vi "encoder_test_3mode_2motor_v3.vi"() -> ()   [LabVIEW 2014]
uses:
  <vilib>/rvi/FXPMathLib/FxpSinAndCos/subVIs/nifxpmath_SinAndCos_SimConfig.ctl
  <vilib>/rvi/Emulation/niFpgaGetClockAttributes.vi
  <vilib>/rvi/Emulation/niFpgaSctlEmulationGetInTimedLoop.vi
  <vilib>/rvi/Emulation/niFpgaEmulationReportErrorSimple.vi
  <vilib>/rvi/eio/common/nirviEmuTemplateMethod_errors.vi
  <vilib>/rvi/Emulation/niFpgaProcessEmulError.vi
  <vilib>/rvi/Emulation/niFpgaCriticalErrorInLSC.vi
  <vilib>/rvi/FXPMathLib/FxpSinAndCos/simVIs/DllFxpSinAndCosTemp_sub.vi
  <vilib>/rvi/interface/RandomDataEmulation/nirviRandomDataMultiElementFPGAFIFO.vi
  <instcachedir>/0/nirviRandomDataMultiElementFPGAFIFO_AD0CFC12EF974623A9C2E4184BC062B2.lvgen/nirviRandomDataMultiElementFPGAFIFO_AD0CFC12EF974623A9C2E4184BC062B2_020.vi
  <vilib>/rvi/interface/RandomDataEmulation/niFpgaRandomDataHandleErrors.vi
  <vilib>/eio/EIONode/EIONode.xnode
  <vilib>/rvi/FXPMathLib/FxpMul/XNode/nifxpmath_Multiplier.xnode
  <vilib>/rvi/FXPMathLib/FxpSinAndCos/XNode/nifxpmath_SinAndCos.xnode
  <vilib>/rvi/Analysis/measure/butterworth/XNode/niFpgaButterworthFilter.xnode
  <vilib>/rvi/FXPMathLib/FxpSub/XNode/nifxpmath_Sub.xnode
  <vilib>/rvi/FXPMathLib/FxpAdd/XNode/nifxpmath_Add.xnode
  <vilib>/rvi/DataTransferAndStorage/Container/XNode/niFpgaContainer.xnode
  <vilib>/rvi/interface/RandomDataEmulation/nirviRandomDataFpgaMultiElementTemplate.vi
  <vilib>/rvi/FXPMathLib/sim/FxpSim.dll
panel:
  out "Dyr_sin_dd":fxp<+/-,64,25>
  out "Dyr_sin_d":fxp<+/-,64,16>
  out "Dyr_sin":fxp<+/-,30,11>
  in  "Sin offset_y":fxp<+/-,29,10>
  out "Sin omega_y":fxp<+/-,41,8>
  in  "Sin magnitude_y":fxp<+/-,11,8>
  in  "Sin wave frequency_y (Hz)":fxp<+/-,21,5>
  out "Dyr_ramp":fxp<+/-,32,7>
  out "Time now_y (s)":fxp<+,52,14>
  out "Dyr_slope":fxp<+/-,32,10>
  in  "Dyr_time":fxp<+/-,32,10>
  in  "Dyr_end":fxp<+/-,32,7>
  out "Dy_i":fxp<+/-,32,16>
  out "Dyr":fxp<+/-,32,7>
  in  "Direction_y":bool
  in  "Command type_y":i16(ring) items=["Step", "Ramp", "Sine"]
  out "Dy_error":fxp<+/-,57,33>
  out "Fmr_y":fxp<+/-,64,50>
  in  "Ki_y":fxp<+/-,16,1>
  in  "Dy_tolorence":fxp<+/-,18,1>
  in  "Kd_y":fxp<+/-,16,1>
  in  "Kp_y":fxp<+/-,16,1>
  in  "scaled coefficients_Dy_dd":i32[](array[numeric])=[780119100, 146811362]
  out "Dy_dd":fxp<+/-,36,47>
  out "va_y":fxp<+/-,36,7>
  out "vb_y":fxp<+/-,37,8>
  out "vd_y":fxp<+/-,20,5>
  out "vq_y":fxp<+/-,20,5> format="%.57g"
  in  "Stop motor_y":bool
  out "Dy_d (mm/s)":fxp<+,64,32>
  out "omega_y (rad/s)":fxp<+/-,64,35>
  in  "Velocity Estimation_y":i16(ring) items=["Step", "Ramp", "Sine"]
  out "Dy_d (T)":fxp<+/-,46,10>
  out "mt 2":u32
  out "omega_y (T)":fxp<+/-,20,9>
  out "omega_y (M)":fxp<+/-,64,30>
  out "Dy_d (M)":fxp<+/-,64,27>
  in  "Dy_d_M_Tc (mSec)":u32 format="%#_6f"
  out "omega_y(M_avg)":fxp<+/-,64,35>
  out "Dy_d (M_avg)":fxp<+,64,32>
  in  "Dy_d_M_avg_Tc (uSec)":u32 caption="Count(uSec)"
  out "rad_y(NrTheta)":fxp<+/-,48,33>
  out "Dy (mm)":fxp<+/-,56,32>
  out "Encoder Position_y":i32
  in  "Encoder Reset_y":bool
  out "omega_p (M_avg)":fxp<+/-,64,35>
  out "Dp_d (M_avg)":fxp<+/-,64,32>
  in  "Dp_d_M_avg_Tc (uSec)":u32 caption="D_d_M_avg_Tc (uSec)"
  out "omega_p (M)":fxp<+/-,64,30>
  out "Dp_d (M)":fxp<+/-,64,27>
  in  "Dp_d_M_Tc (mSec)":u32 format="%#_6f"
  out "Dp_d (T)":fxp<+/-,46,10>
  out "omega_p(T)":fxp<+/-,20,9>
  in  "Velocity Estimation_p":i16(ring) items=["M_avg method", "M method", "T method"]
  out "Dpr_ramp":fxp<+/-,64,30>
  out "Dpr_slope":fxp<+/-,32,10>
  in  "Dpr_time":fxp<+/-,32,10>
  out "Dpr_sin":fxp<+/-,30,11>
  out "Dpr_sin_d":fxp<+/-,64,16>
  out "Dpr_sin_dd":fxp<+/-,64,25>
  out "Sin omega_p":fxp<+/-,41,8>
  in  "Sin offset_p":fxp<+/-,27,10>
  in  "Sin magnitude_p":fxp<+/-,11,8>
  in  "Sin wave frequency_p (Hz)":fxp<+/-,21,5>
  out "Time now_p (s)":fxp<+,52,14>
  out "Dpr":fxp<+/-,64,31>
  in  "Dpr_end":fxp<+/-,22,7>
  in  "Command type_p":i16(ring) items=["Step", "Ramp", "Sine"]
  out "Dp_i":fxp<+/-,34,18>
  in  "Dp_tolorence":fxp<+/-,18,1>
  in  "Ki_p":fxp<+/-,20,6>
  out "Dp_error":fxp<+/-,24,11>
  in  "Direction_p":bool
  out "Fmr_p":fxp<+/-,64,31>
  in  "Kd_p":fxp<+/-,20,8>
  in  "Kp_p":fxp<+/-,20,12>
  in  "scaled coefficients_Dp_dd":i32[](array[numeric])=[780119100, 146811362]
  out "Dp_dd":fxp<+/-,36,29>
  in  "Ini coe.":bool
  out "va_p":fxp<+/-,38,8>
  out "vb_p":fxp<+/-,38,8>
  in  "Stop motor_p":bool
  out "vq_p":fxp<+/-,20,5> format="%.57g"
  out "vd_p":fxp<+/-,20,5>
  out "Dp_d (mm/s)":fxp<+/-,32,12>
  out "mt":u32
  out "omega_p (rad/s)":fxp<+/-,32,18>
  in  "mt0":u32
  out "Dp (mm)":fxp<+/-,22,7>
  out "rad_p(NrTheta)":fxp<+/-,33,18>
  out "Encoder Position_p":i32
  in  "Encoder Reset_p":bool
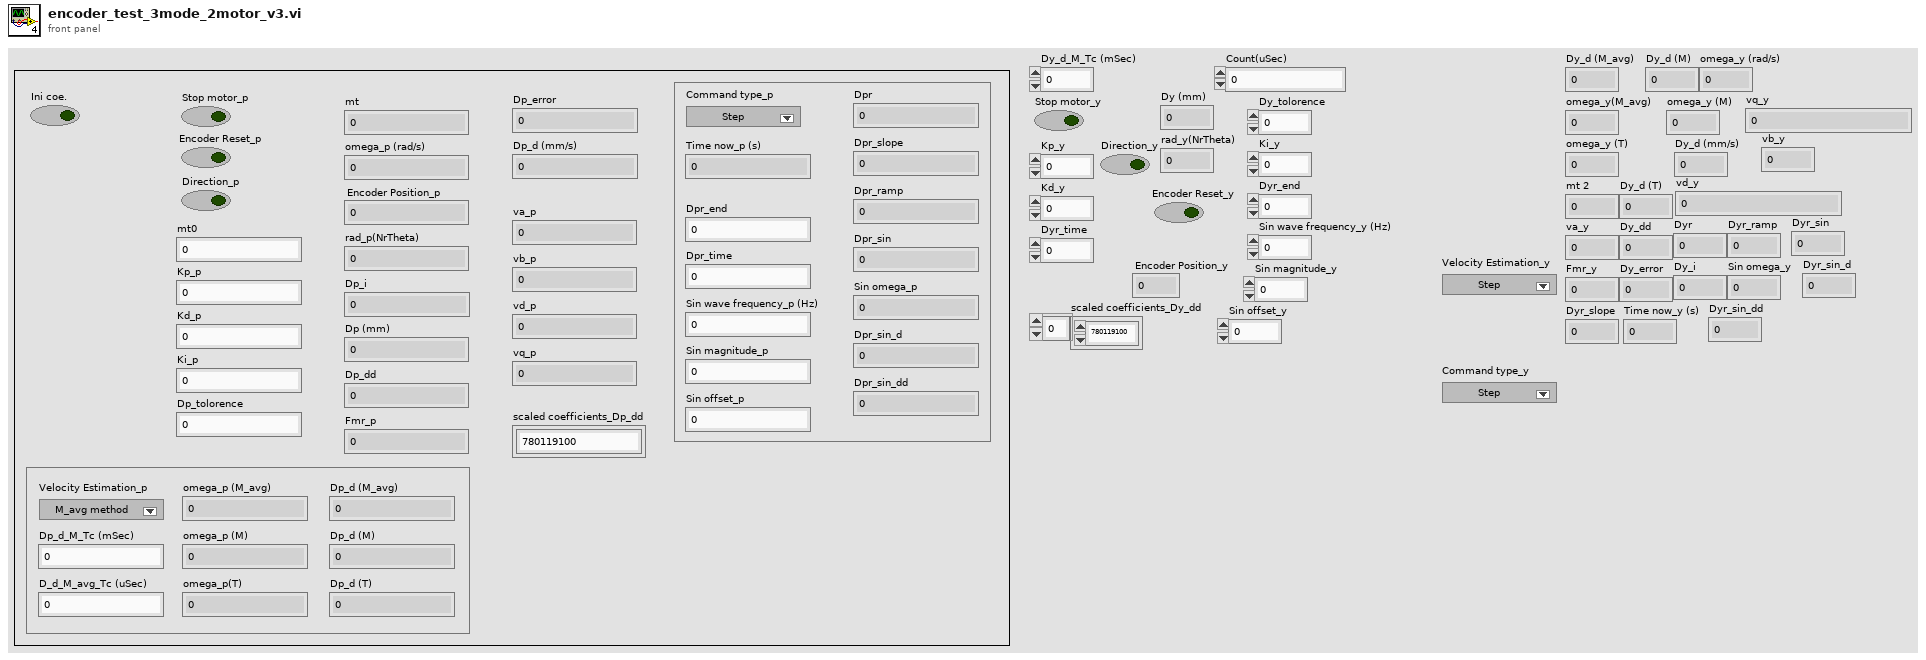
[diagram p1: front panel]
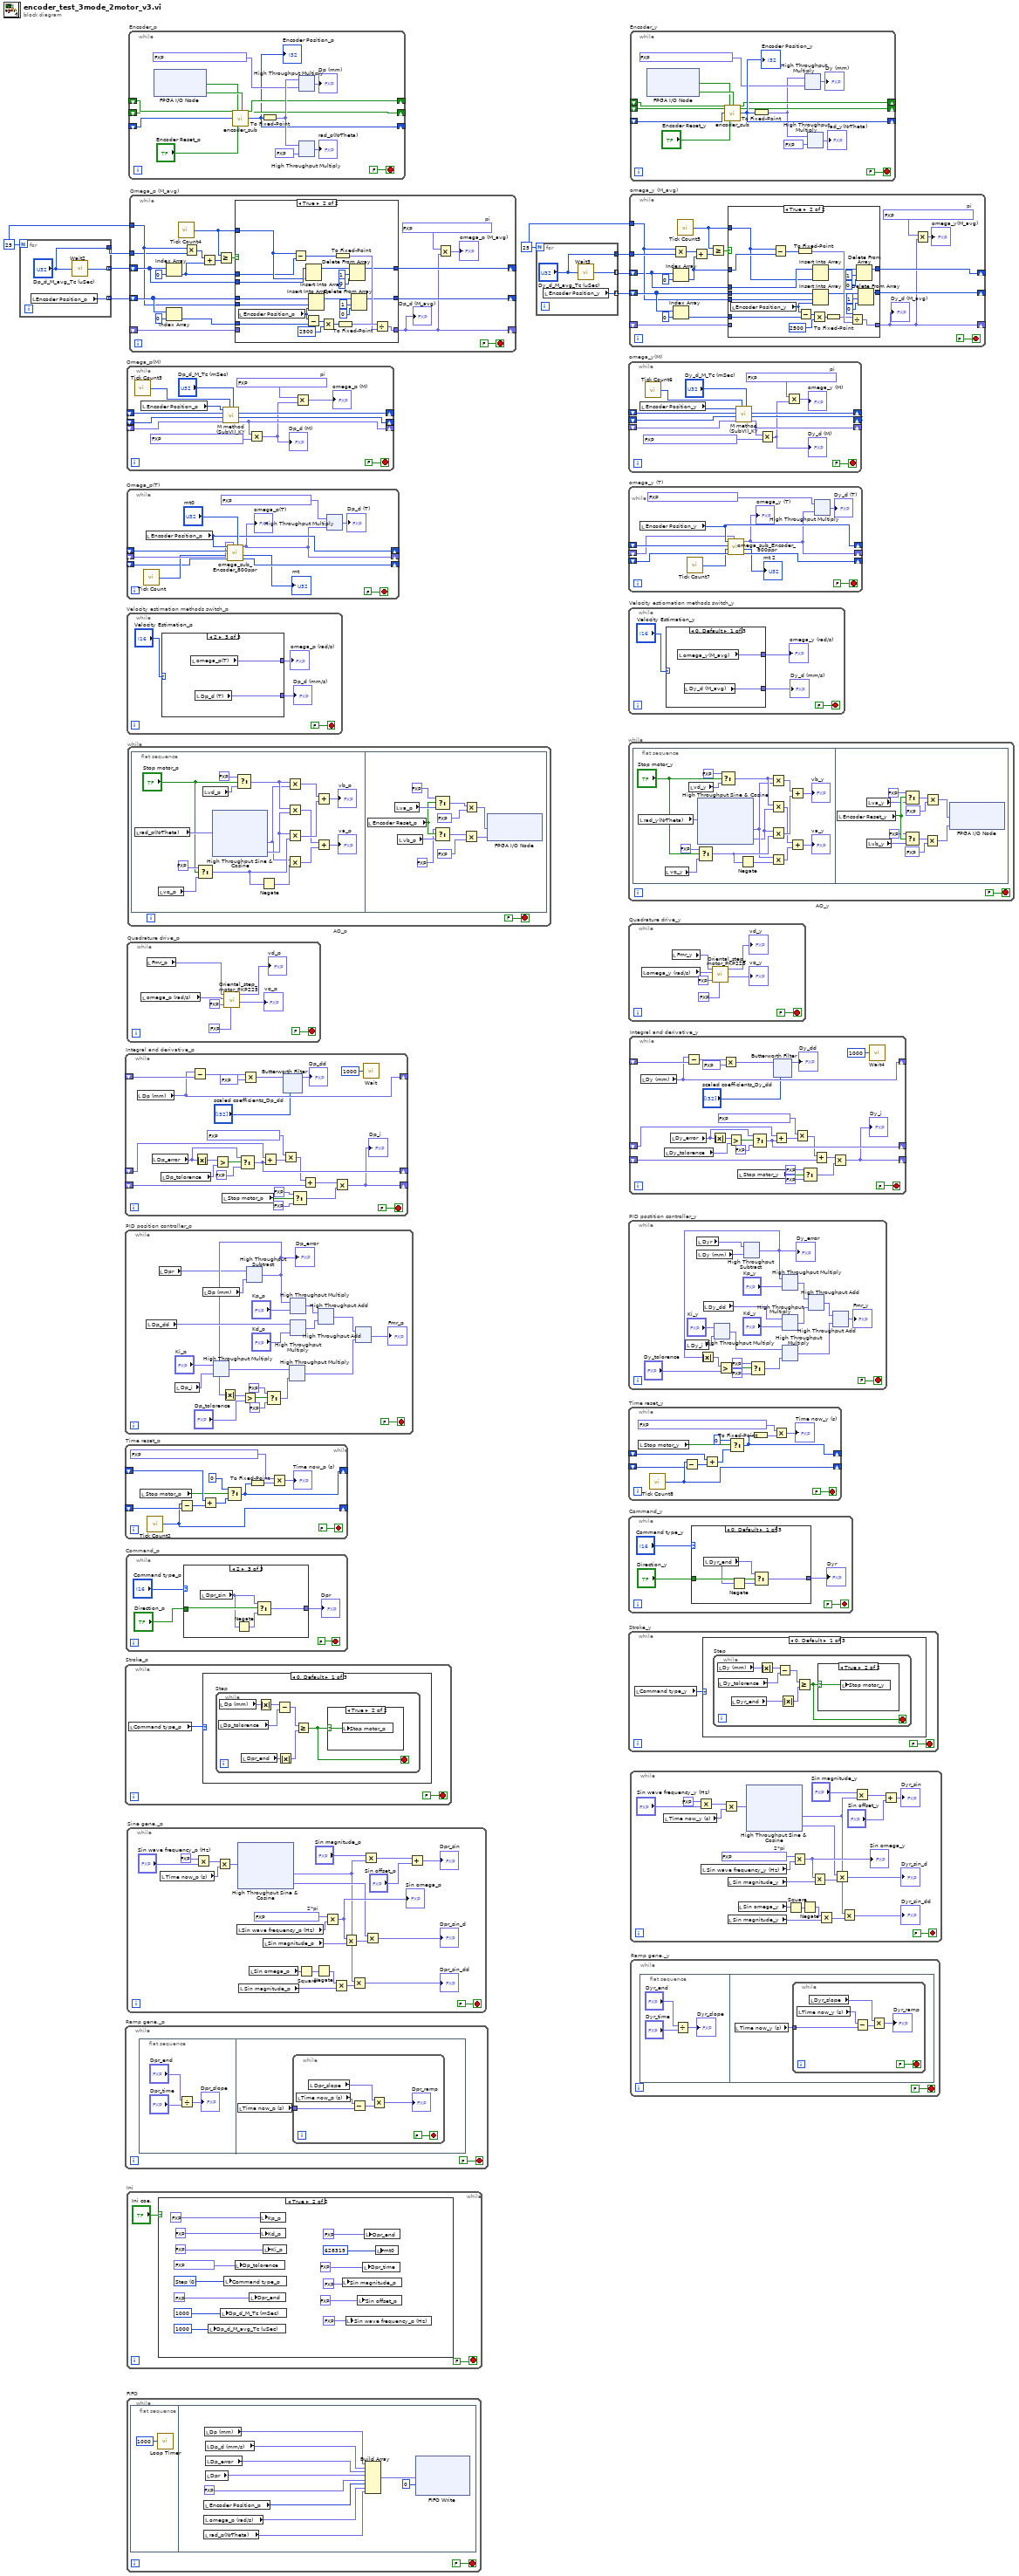
[diagram p0: block diagram]
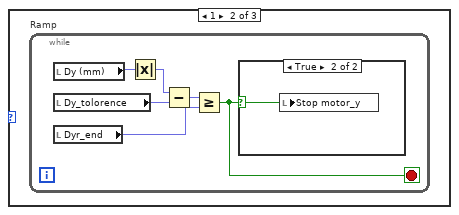
[diagram p3: hidden frame]
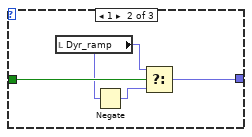
[diagram p6: hidden frame]
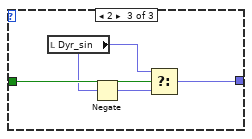
[diagram p7: hidden frame]
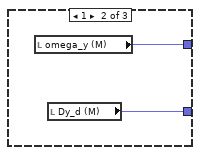
[diagram p8: hidden frame]
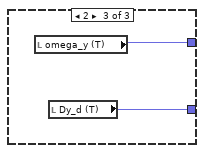
[diagram p9: hidden frame]
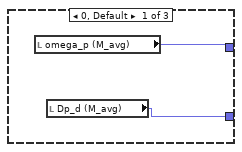
[diagram p12: hidden frame]
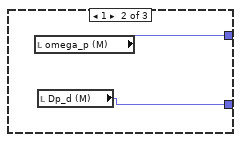
[diagram p13: hidden frame]
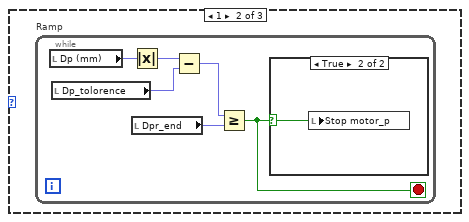
[diagram p15: hidden frame]
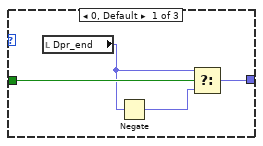
[diagram p18: hidden frame]
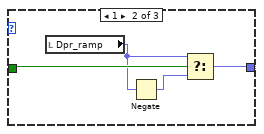
[diagram p19: hidden frame]
diagram:
  w4 = 25
  w8 = 25
  n1 = for {
    N: w8 -> [_]
    tunnel: ["Dp_d_M_avg_Tc (uSec)"] -> w5
    tunnel: [w10] -> w7 mode=indexing
    tunnel: [w9] -> w6 mode=indexing
    n2 = local read "Encoder Position_p"() -> (w9:i32)
    n3 = call "Wait2"("Count(uSec)"="Dp_d_M_avg_Tc (uSec)") -> ("Tick Count(uSec)"=w10:u32)
  }
  n4 = while "Integral and derivative_p" {
    shift-right: [w32] -> _
    shift-left: _ -> [w36]
    shift-right: [w22] -> _
    shift-left: _ -> [w23]
    shift-right: [w12] -> _
    shift-left: _ -> [w16]
    stop <- FALSE stop-if-true
    n5 = local read "Dp (mm)"() -> (w32:fxp<+/-,22,7>)
    n6 = local read "Dp_error"() -> (w24:fxp<+/-,24,11>)
    n7 = local read "Dp_tolorence"() -> (w27:fxp<+/-,18,1>)
    n8 = Subtract(x=w32, y=w36) -> (x-y=w35:fxp<+/-,23,8>)
    n9 = Absolute Value(x=w24) -> (abs(x)=w28:fxp<+,24,11>)
    n10 = Greater?(x=w28, y=w27) -> (0:w26:bool)
    n11 = local read "Stop motor_p"() -> (w19:bool)
    n12 = Select(t=w24, s=w26, f=fxp<+,24,11> 0.0) -> (s? t:f=w22:fxp<+/-,25,12>)
    n13 = Multiply(x=w35, y=fxp<+/-,33,13> 1000.0) -> (x*y=w33:fxp<+/-,55,20>)
    n14 = Add(x=w23, y=w22) -> (x+y=w21:fxp<+/-,26,13>)
    n15 = Multiply(x=fxp<+/-,30,12> 0.000499725341796875, y=w21) -> (x*y=w15:fxp<+/-,55,24>)
    n16 = xnode "Butterworth Filter"("input data"=w33, "scaled coefficients"="scaled coefficients_Dp_dd") -> ("output data"=→"Dp_dd":fxp<+/-,36,24>)  [unwired: 1 in]
    n17 = Select(t=fxp<+,1,1> 0.0, s=w19, f=fxp<+,1,1> 1.0) -> (s? t:f=w13:fxp<+,1,1>)
    n18 = Add(x=w15, y=w16) -> (x+y=w14:fxp<+/-,32,16>)
    n19 = Multiply(x=w14, y=w13) -> (x*y=w12:fxp<+/-,32,16>)
    "Dp_i" <- w12
    n20 = call "Wait"("Count(uSec)"=u32 1000) -> ()  [unwired: 1 out]
  }
  n21 = while "PID position controller_p" {
    stop <- FALSE stop-if-true
    n22 = local read "Dp_dd"() -> (w62:fxp<+/-,36,29>)
    n23 = local read "Dpr"() -> (w46:fxp<+/-,64,31>)
    n24 = local read "Dp_i"() -> (w57:fxp<+/-,34,18>)
    n25 = local read "Dp (mm)"() -> (w66:fxp<+/-,22,7>)
    n26 = xnode ("High Throughput Multiply")("x"="Ki_p", "y"=w57) -> ("x*y"=w51:fxp<+/-,54,24>)
    n27 = xnode "High Throughput Subtract"("x"=w46, "y"=w66) -> ("x-y"=w55:fxp<+/-,64,32>)
    "Dp_error" <- w55
    n28 = Absolute Value(x=w55) -> (abs(x)=w56:fxp<+,64,32>)
    n29 = Greater?(x=w56, y="Dp_tolorence") -> (0:w54:bool)
    n30 = Select(t=fxp<+,10,2> 1.0, s=w54, f=fxp<+,10,2> 0.0) -> (s? t:f=w50:fxp<+,10,2>)
    n31 = xnode ("High Throughput Multiply")("x"=w51, "y"=w50) -> ("x*y"=w47:fxp<+/-,64,26>)
    n32 = xnode ("High Throughput Multiply")("x"=w55, "y"="Kp_p") -> ("x*y"=w64:fxp<+/-,64,44>)
    n33 = xnode ("High Throughput Multiply")("x"=w62, "y"="Kd_p") -> ("x*y"=w63:fxp<+/-,56,37>)
    n34 = xnode ("High Throughput Add")("x"=w64, "y"=w63) -> ("x+y"=w48:fxp<+/-,64,45>)
    n35 = xnode ("High Throughput Add")("x"=w48, "y"=w47) -> ("x+y"=→"Fmr_p":fxp<+/-,64,46>)
  }
  n36 = while "Time reset_p" {
    shift-right: [w70] -> _
    shift-left: _ -> [w77]
    shift-right: [w72] -> _
    shift-left: _ -> [w73]
    stop <- FALSE stop-if-true
    n37 = local read "Stop motor_p"() -> (w75:bool)
    n38 = call "Tick Count2"() -> ("Tick Count(uSec)"=w72:u32)
    n39 = Subtract(x=w72, y=w73) -> (x-y=w78:u32)
    n40 = Add(x=w77, y=w78) -> (x+y=w76:u32)
    n41 = Select(t=u32 0, s=w75, f=w76) -> (s? t:f=w70:u32)
    n42 = To Fixed-Point(number=w70) -> (fixed-point=w69:fxp<+,32,32>)  [unwired: 1 in]
    n43 = Multiply(x=fxp<+,20,-18> 1.0000003385357559e-06, y=w69) -> (x*y=→"Time now_p (s)":fxp<+,52,14>)
  }
  n44 = while "Stroke_p" {
    stop <- FALSE stop-if-true
    n45 = local read "Command type_p"() -> (w80:i16)
    n46 = case shown="0, Default" w80 {
      frame 0, Default {
        n47 = while "Step" {
          stop <- w81 stop-if-true
          n48 = local read "Dp_tolorence"() -> (w83:fxp<+/-,18,1>)
          n49 = local read "Dp (mm)"() -> (w85:fxp<+/-,22,7>)
          n50 = local read "Dpr_end"() -> (w87:fxp<+/-,22,7>)
          n51 = Absolute Value(x=w85) -> (abs(x)=w84:fxp<+,22,7>)
          n52 = Subtract(x=w84, y=w83) -> (x-y=w82:fxp<+/-,25,8>)
          n53 = Absolute Value(x=w87) -> (abs(x)=w86:fxp<+,22,7>)
          n54 = Greater Or Equal?(x=w82, y=w86) -> (x >= y?=w81:bool)
          n55 = case shown="True" w81 {
            selector: w81 -> [_ w88]
            frame False {
            }
            frame True {
              n56 = local write "Stop motor_p"(w88) -> ()
            }
          }
        }
      }
      frame 1 {
        n57 = while "Ramp" {
          stop <- w89 stop-if-true
          n58 = local read "Dp (mm)"() -> (w91:fxp<+/-,22,7>)
          n59 = local read "Dp_tolorence"() -> (w93:fxp<+/-,18,1>)
          n60 = Absolute Value(x=w91) -> (abs(x)=w92:fxp<+,22,7>)
          n61 = local read "Dpr_end"() -> (w90:fxp<+/-,22,7>)
          n62 = Subtract(x=w92, y=w93) -> (x-y=w94:fxp<+/-,25,8>)
          n63 = Greater Or Equal?(x=w94, y=w90) -> (x >= y?=w89:bool)
          n64 = case shown="True" w89 {
            selector: w89 -> [_ w95]
            frame False {
            }
            frame True {
              n65 = local write "Stop motor_p"(w95) -> ()
            }
          }
        }
      }
      frame 2 {
      }
    }
  }
  n66 = while "Ramp gene._p" {
    stop <- FALSE stop-if-true
    n67 = flat-sequence {
      frame #0 {
        n68 = Divide(x="Dpr_end", y="Dpr_time") -> (x/y=→"Dpr_slope":fxp<+/-,55,30>)
      }
      frame #1 {
        n69 = local read "Time now_p (s)"() -> (w100:fxp<+,52,14>)
        n70 = while {
          tunnel: w100 -> [w106]
          stop <- FALSE stop-if-true
          n71 = local read "Time now_p (s)"() -> (w103:fxp<+,52,14>)
          n72 = local read "Dpr_slope"() -> (w104:fxp<+/-,32,10>)
          n73 = Subtract(x=w103, y=w106) -> (x-y=w105:fxp<+/-,53,15>)
          n74 = Multiply(x=w104, y=w105) -> (x*y=→"Dpr_ramp":fxp<+/-,64,24>)
        }
      }
    }
  }
  n75 = while "Command_p" {
    stop <- FALSE stop-if-true
    n76 = case shown="2" "Command type_p" {
      tunnel: [w111 w115 w119] -> w109
      tunnel: "Direction_p" -> [w114 w118 w122]
      frame 0, Default {
        n77 = local read "Dpr_end"() -> (w113:fxp<+/-,22,7>)
        n78 = Negate(x=w113) -> (-x=w112:fxp<+/-,23,8>)
        n79 = Select(t=w113, s=w114, f=w112) -> (s? t:f=w111:fxp<+/-,23,8>)
      }
      frame 1 {
        n80 = local read "Dpr_ramp"() -> (w116:fxp<+/-,64,30>)
        n81 = Negate(x=w116) -> (-x=w117:fxp<+/-,64,31>)
        n82 = Select(t=w116, s=w118, f=w117) -> (s? t:f=w115:fxp<+/-,64,31>)
      }
      frame 2 {
        n83 = local read "Dpr_sin"() -> (w120:fxp<+/-,30,11>)
        n84 = Negate(x=w120) -> (-x=w121:fxp<+/-,29,10>)
        n85 = Select(t=w120, s=w122, f=w121) -> (s? t:f=w119:fxp<+/-,30,11>)
      }
    }
    "Dpr" <- w109
  }
  n86 = while "Omega_p(M)" {
    shift-right: [w134] -> _
    shift-left: _ -> [w135]
    shift-right: [w130] -> _
    shift-left: _ -> [w131]
    shift-right: [w128] -> _
    shift-left: _ -> [w129]
    stop <- FALSE stop-if-true
    w125 = fxp<+/-,27,3> 3.1415926218032837  # pi
    n87 = call "Tick Count3"() -> ("Tick Count(mSec)"=w133:u32)
    n88 = local read "Encoder Position_p"() -> (w136:i32)
    n89 = call "M method (SubVI)_KY.vi"("Tc (mSec)"="Dp_d_M_Tc (mSec)", "Tick Count (mSec)"=w133, "Encoder velocity_pre (pulse/s)"=w129, "Shift Register in 2"=w131, "Shift Register in 1"=w135, "Encoder pulses"=w136) -> ("Encoder velocity (pulse/s)"=w128:fxp<+/-,64,32>, "Shift Register out 2"=w130:i32, "Shift Register out 1"=w134:u32)  [unwired: 3 in]
    n90 = Multiply(x=w128, y=fxp<+/-,20,-5> 0.002499997615814209) -> (x*y=w126:fxp<+/-,64,27>)
    "Dp_d (M)" <- w126
    n91 = Multiply(x=w125, y=w126) -> (x*y=→"omega_p (M)":fxp<+/-,64,30>)
  }
  n92 = while "Omega_p(T)" {
    shift-right: [w146] -> _
    shift-left: _ -> [w147]
    shift-right: [w139] -> _
    shift-left: _ -> [w145]
    shift-right: [w142] -> _
    shift-left: _ -> [w143]
    stop <- FALSE stop-if-true
    n93 = call "Tick Count"() -> ("Tick Count(Ticks)"=w144:u32)
    n94 = local read "Encoder Position_p"() -> (w146:i32)
    n95 = call "omega_sub_Encoder_800ppr.vi"("mt0"="mt0", "omega_pre"=w145, "ticks_m_pre"=w143, "ticks"=w144, "count_pre"=w147, "count"=w146) -> ("ticks_m"=w142:u32, "mt"=→"mt":u32, "omega"=w139:fxp<+/-,20,9>)  [unwired: 3 in]
    "omega_p(T)" <- w139
    n96 = xnode ("High Throughput Multiply")("x"=fxp<+/-,26,1> 0.3183099031448364, "y"=w139) -> ("x*y"=→"Dp_d (T)":fxp<+/-,46,10>)
  }
  n97 = while "Velocity estimation methods switch_p" {
    stop <- FALSE stop-if-true
    n98 = case shown="2" "Velocity Estimation_p" {
      tunnel: [w154 w156 w158] -> w151
      tunnel: [w153 w155 w157] -> w150
      frame 0, Default {
        n99 = local read "omega_p (M_avg)"() -> (w154:fxp<+/-,64,35>)
        n100 = local read "Dp_d (M_avg)"() -> (w153:fxp<+/-,64,32>)
      }
      frame 1 {
        n101 = local read "omega_p (M)"() -> (w156:fxp<+/-,64,30>)
        n102 = local read "Dp_d (M)"() -> (w155:fxp<+/-,64,27>)
      }
      frame 2 {
        n103 = local read "omega_p(T)"() -> (w158:fxp<+/-,20,9>)
        n104 = local read "Dp_d (T)"() -> (w157:fxp<+/-,46,10>)
      }
    }
    "Dp_d (mm/s)" <- w150
    "omega_p (rad/s)" <- w151
  }
  n105 = while "Ini" {
    stop <- FALSE stop-if-true
    n106 = case shown="True" "Ini coe." {
      frame False {
      }
      frame True {
        w168 = i16 0 items=["Step", "Ramp", "Sine"] ("Command type")
        n107 = local write "Dp_d_M_avg_Tc (uSec)"(u32 1000 ("D_d_M_avg_Tc (uSec)")) -> ()
        n108 = local write "Dp_d_M_Tc (mSec)"(u32 1000 ("D_d_M_Tc (uSec)")) -> ()
        n109 = local write "Command type_p"(w168) -> ()
        n110 = local write "Dp_tolorence"(fxp<+/-,14,3> 0.009765625 ("D_tolorence")) -> ()
        n111 = local write "Dpr_end"(fxp<+/-,16,11> 20.0 ("Dr_end")) -> ()
        n112 = local write "Kp_p"(fxp<+/-,20,12> 10.0 ("Kp")) -> ()
        n113 = local write "Kd_p"(fxp<+/-,20,8> 2.0 ("Kd")) -> ()
        n114 = local write "Ki_p"(fxp<+/-,20,6> 8.0 ("D_i")) -> ()
        n115 = local write "Sin magnitude_p"(fxp<+/-,11,8> 20.0 ("Sin magnitude")) -> ()
        n116 = local write "Sin wave frequency_p (Hz)"(fxp<+/-,21,5> 0.5 ("Sin wave frequency (Hz)")) -> ()
        n117 = local write "Sin offset_p"(fxp<+/-,27,10> 0.0 ("Sin offset")) -> ()
        n118 = local write "Dpr_time"(fxp<+/-,16,11> 5.0 ("Dr_time")) -> ()
        n119 = local write "Dpr_end"(fxp<+/-,11,7> 20.0 ("Fmr")) -> ()
        n120 = local write "mt0"(u32 628319 ("mt0")) -> ()
      }
    }
  }
  n121 = while "FIFO" {
    stop <- FALSE stop-if-true
    n122 = flat-sequence {
      frame #0 {
        n123 = call "Loop Timer"("Count(uSec)"=u32 1000) -> ()  [unwired: 1 out]
      }
      frame #1 {
        n124 = local read "Encoder Position_p"() -> (w180:i32)
        n125 = local read "omega_p (rad/s)"() -> (w179:fxp<+/-,32,18>)
        n126 = local read "rad_p(NrTheta)"() -> (w178:fxp<+/-,33,18>)
        n127 = local read "Dp (mm)"() -> (w184:fxp<+/-,22,7>)
        n128 = local read "Dp_d (mm/s)"() -> (w183:fxp<+/-,32,12>)
        n129 = local read "Dp_error"() -> (w182:fxp<+/-,24,11>)
        n130 = local read "Dpr"() -> (w181:fxp<+/-,64,31>)
        n131 = Build Array(w184, w183, w182, w181, fxp<+/-,64,32> 0.0 ("element"), w180, w179, w178) -> (w185:fxp<+/-,64,32>[])
        n132 = xnode ("FIFO Write")("Element"=w185, "Timeout"=0) -> ()  [unwired: 1 in, 2 out]
      }
    }
  }
  n133 = while "Quadrature drive_p" {
    stop <- FALSE stop-if-true
    n134 = local read "omega_p (rad/s)"() -> (w189:fxp<+/-,32,18>)
    n135 = local read "Fmr_p"() -> (w187:fxp<+/-,64,31>)
    n136 = call "Oriental_step_motor_PKP225.vi"("F_Threshold"=fxp<+,12,12> 10.0, "dFmr"=fxp<+/-,25,15> 0.0, "omega"=w189, "Fmr"=w187) -> ("vq_F"=→"vq_p":fxp<+/-,20,5>, "vd_F"=→"vd_p":fxp<+/-,20,5>)  [unwired: 6 in]
  }
  n137 = while "Sine gene._p" {
    stop <- FALSE stop-if-true
    w211 = fxp<+,20,3> 6.2831878662109375  # 2*pi
    n138 = local read "Time now_p (s)"() -> (w214:fxp<+,52,14>)
    n139 = Multiply(x=fxp<+,1,2> 2.0, y="Sin wave frequency_p (Hz)") -> (x*y=w215:fxp<+/-,21,6>)
    n140 = Multiply(x=w215, y=w214) -> (x*y=w195:fxp<+/-,64,20>)
    n141 = local read "Sin wave frequency_p (Hz)"() -> (w210:fxp<+/-,21,5>)
    n142 = xnode "High Throughput Sine & Cosine"("x (pi)"=w195) -> ("sin(x)"=w199:fxp<+/-,18,2>, "cos(x)"=w206:fxp<+/-,18,2>)
    n143 = local read "Sin magnitude_p"() -> (w201:fxp<+/-,11,8>)
    n144 = local read "Sin omega_p"() -> (w202:fxp<+/-,41,8>)
    n145 = local read "Sin magnitude_p"() -> (w205:fxp<+/-,11,8>)
    n146 = Square(x=w202) -> (x^2=w203:fxp<+,64,14>)
    n147 = Negate(x=w203) -> (-x=w200:fxp<+/-,64,15>)
    n148 = Multiply(x=w211, y=w210) -> (x*y=w207:fxp<+/-,41,8>)
    "Sin omega_p" <- w207
    n149 = Multiply(x=w200, y=w201) -> (x*y=w204:fxp<+/-,64,23>)
    n150 = Multiply(x=w207, y=w205) -> (x*y=w212:fxp<+/-,51,15>)
    n151 = Multiply(x=w199, y=w204) -> (x*y=→"Dpr_sin_dd":fxp<+/-,64,25>)
    n152 = Multiply(x="Sin magnitude_p", y=w199) -> (x*y=w213:fxp<+/-,29,10>)
    n153 = Multiply(x=w206, y=w212) -> (x*y=→"Dpr_sin_d":fxp<+/-,64,16>)
    n154 = Add(x=w213, y="Sin offset_p") -> (x+y=→"Dpr_sin":fxp<+/-,30,11>)
  }
  n155 = while "AO_p" {
    stop <- FALSE stop-if-true
    n156 = flat-sequence {
      frame #0 {
        n157 = local read "rad_p(NrTheta)"() -> (w264:fxp<+/-,33,18>)
        n158 = local read "vq_p"() -> (w262:fxp<+/-,20,5>)
        n159 = Select(t=fxp<+,20,5> 0.0, s="Stop motor_p", f=w262) -> (s? t:f=w259:fxp<+/-,21,6>)
        n160 = local read "vd_p"() -> (w263:fxp<+/-,20,5>)
        n161 = xnode "High Throughput Sine & Cosine"("x (pi)"=w264) -> ("sin(x)"=w255:fxp<+/-,17,2>, "cos(x)"=w257:fxp<+/-,17,2>)
        n162 = Select(t=fxp<+,20,5> 0.0, s="Stop motor_p", f=w263) -> (s? t:f=w256:fxp<+/-,21,6>)
        n163 = Negate(x=w259) -> (-x=w258:fxp<+/-,21,6>)
        n164 = Multiply(x=w256, y=w255) -> (x*y=w254:fxp<+/-,37,7>)
        n165 = Multiply(x=w256, y=w257) -> (x*y=w252:fxp<+/-,37,7>)
        n166 = Multiply(x=w257, y=w259) -> (x*y=w253:fxp<+/-,37,7>)
        n167 = Multiply(x=w255, y=w258) -> (x*y=w251:fxp<+/-,37,7>)
        n168 = Add(x=w254, y=w253) -> (x+y=→"vb_p":fxp<+/-,38,8>)
        n169 = Add(x=w252, y=w251) -> (x+y=→"va_p":fxp<+/-,38,8>)
      }
      frame #1 {
        n170 = local read "Encoder Reset_p"() -> (w298:bool)
        n171 = local read "va_p"() -> (w300:fxp<+/-,38,8>)
        n172 = local read "vb_p"() -> (w299:fxp<+/-,38,8>)
        n173 = Select(t=fxp<+/-,20,5> 5.0 ("y"), s=w298, f=w300) -> (s? t:f=w301:fxp<+/-,38,8>)
        n174 = Select(t=fxp<+/-,20,5> 0.0 ("y"), s=w298, f=w299) -> (s? t:f=w302:fxp<+/-,38,8>)
        n175 = Multiply(x=w302, y=fxp<+/-,20,5> -0.5) -> (x*y=w306:fxp<+/-,57,12>)
        n176 = Multiply(x=w301, y=fxp<+/-,20,5> -0.5) -> (x*y=w305:fxp<+/-,57,12>)
        n177 = xnode "FPGA I/O Node"("Mod8/AO0"=w305, "Mod8/AO1"=w306) -> ()  [unwired: 2 in, 2 out]
      }
    }
  }
  n178 = while "Encoder_p" {
    shift-right: [w313] -> _
    shift-left: _ -> [w315]
    shift-right: [w312] -> _
    shift-left: _ -> [w314]
    shift-right: [w310] -> _
    shift-left: _ -> [w311]
    stop <- FALSE stop-if-true
    n179 = xnode "FPGA I/O Node"() -> ("Mod4/DI3"=w320:bool, "Mod4/DI4"=w321:bool)  [unwired: 2 in, 2 out]
    n180 = call "encoder_sub.vi"("A_pre"=w315, "B_pre"=w314, "Encoder Position_pre"=w311, "A input"=w320, "Encoder Position Reset"="Encoder Reset_p", "B input"=w321) -> ("A"=w313:bool, "B"=w312:bool, "Encoder Position (Counts)"=w310:i32)  [unwired: 19 in]
    "Encoder Position_p" <- w310
    n181 = To Fixed-Point(number=w310) -> (fixed-point=w318:fxp<+/-,32,32>)  [unwired: 1 in]
    n182 = xnode ("High Throughput Multiply")("x"=w318, "y"=fxp<+/-,24,0> 0.002499997615814209) -> ("x*y"=→"Dp (mm)":fxp<+/-,56,32>)
    n183 = xnode ("High Throughput Multiply")("x"=w318, "y"=fxp<+/-,24,0> 0.125) -> ("x*y"=→"rad_p(NrTheta)":fxp<+/-,56,32>)
  }
  n184 = while "Omega_p (M_avg)" {
    tunnel: w8 -> [w333]
    shift-right: [w326] -> _
    shift-left: w7 -> [w337]
    shift-right: [w325] -> _
    shift-left: _ -> [w328]
    shift-right: [w327] -> _
    shift-left: w6 -> [w336]
    tunnel: w5 -> [w330]
    stop <- FALSE stop-if-true
    w324 = fxp<+/-,27,3> 3.1415926218032837  # pi
    n185 = Index Array(array=w337, index=0) -> (element=w331:u32)
    n186 = Index Array(array=w336, index=0) -> (element=w332:i32)
    n187 = call "Tick Count4"() -> ("Tick Count(uSec)"=w334:u32)
    n188 = Multiply(x=w333, y=w330) -> (x*y=w338:u32)
    n189 = Add(x=w338, y=w331) -> (x+y=w335:u32)
    n190 = Greater Or Equal?(x=w334, y=w335) -> (x >= y?=w329:bool)
    n191 = case shown="True" w329 {
      tunnel: w337 -> [w343 w360]
      tunnel: w336 -> [w342 w359]
      tunnel: w334 -> [_ w352]
      tunnel: w333 -> [_ w358]
      tunnel: w332 -> [_ w356]
      tunnel: w331 -> [_ w351]
      tunnel: w328 -> [w341 _]
      tunnel: [w342 w346] -> w327
      tunnel: [w343 w345] -> w326
      tunnel: [w341 w344] -> w325
      frame False {
      }
      frame True {
        n192 = local read "Encoder Position_p"() -> (w357:i32)
        n193 = Subtract(x=w352, y=w351) -> (x-y=w349:u32)
        n194 = Insert Into Array(array=w360, new element=w352) -> (w361:u32[])  [unwired: 1 in]
        n195 = Subtract(x=w357, y=w356) -> (x-y=w355:i32)
        n196 = Insert Into Array(array=w359, index=w358, new element=w357) -> (w362:i32[])
        n197 = Multiply(x=w355, y=2500) -> (x*y=w353:i32)
        n198 = To Fixed-Point(number=w349) -> (fixed-point=w347:fxp<+,32,32>)  [unwired: 1 in]
        n199 = To Fixed-Point(number=w353) -> (fixed-point=w348:fxp<+/-,32,32>)  [unwired: 1 in]
        n200 = Delete From Array(array=w361, length=1, index=0) -> (array with subset deleted=w345:u32[])  [unwired: 1 out]
        n201 = Delete From Array(array=w362, length=1, index=0) -> (array with subset deleted=w346:i32[])  [unwired: 1 out]
        n202 = Divide(x=w348, y=w347) -> (x/y=w344:fxp<+/-,64,32>)
      }
    }
    "Dp_d (M_avg)" <- w325
    n203 = Multiply(x=w324, y=w325) -> (x*y=→"omega_p (M_avg)":fxp<+/-,64,35>)
  }
  n204 = for {
    N: w4 -> [_]
    tunnel: ["Dy_d_M_avg_Tc (uSec)"] -> w3
    tunnel: [w367] -> w1 mode=indexing
    tunnel: [w366] -> w2 mode=indexing
    n205 = local read "Encoder Position_y"() -> (w366:i32)
    n206 = call "Wait3"("Count(uSec)"="Dy_d_M_avg_Tc (uSec)") -> ("Tick Count(uSec)"=w367:u32)
  }
  n207 = while "omega_y(M)" {
    shift-right: [w375] -> _
    shift-left: _ -> [w379]
    shift-right: [w376] -> _
    shift-left: _ -> [w378]
    shift-right: [w374] -> _
    shift-left: _ -> [w377]
    stop <- FALSE stop-if-true
    w371 = fxp<+/-,27,3> 3.1415926218032837  # pi
    n208 = local read "Encoder Position_y"() -> (w382:i32)
    n209 = call "Tick Count6"() -> ("Tick Count(mSec)"=w381:u32)
    n210 = call "M method (SubVI)_KY.vi"("Tc (mSec)"="Dy_d_M_Tc (mSec)", "Tick Count (mSec)"=w381, "Encoder velocity_pre (pulse/s)"=w377, "Shift Register in 2"=w378, "Shift Register in 1"=w379, "Encoder pulses"=w382) -> ("Encoder velocity (pulse/s)"=w374:fxp<+/-,64,32>, "Shift Register out 2"=w376:i32, "Shift Register out 1"=w375:u32)  [unwired: 3 in]
    n211 = Multiply(x=w374, y=fxp<+/-,20,-5> 0.002499997615814209) -> (x*y=w372:fxp<+/-,64,27>)
    "Dy_d (M)" <- w372
    n212 = Multiply(x=w371, y=w372) -> (x*y=→"omega_y (M)":fxp<+/-,64,30>)
  }
  n213 = while "omega_y (T)" {
    shift-right: [w392] -> _
    shift-left: _ -> [w391]
    shift-right: [w386] -> _
    shift-left: _ -> [w390]
    shift-right: [w393] -> _
    shift-left: _ -> [w389]
    stop <- FALSE stop-if-true
    n214 = local read "Encoder Position_y"() -> (w392:i32)
    n215 = call "Tick Count7"() -> ("Tick Count(Ticks)"=w388:u32)
    n216 = call "omega_sub_Encoder_800ppr.vi"("omega_pre"=w390, "ticks_m_pre"=w389, "ticks"=w388, "count_pre"=w391, "count"=w392) -> ("ticks_m"=w393:u32, "mt"=→"mt 2":u32, "omega"=w386:fxp<+/-,20,9>)  [unwired: 4 in]
    "omega_y (T)" <- w386
    n217 = xnode "High Throughput Multiply"("x"=fxp<+/-,26,1> 0.3183099031448364, "y"=w386) -> ("x*y"=→"Dy_d (T)":fxp<+/-,46,10>)
  }
  n218 = while "Velocity estiomation methods switch_y" {
    stop <- FALSE stop-if-true
    n219 = case shown="0, Default" "Velocity Estimation_y" {
      tunnel: [w399 w400 w403] -> w396
      tunnel: [w398 w401 w402] -> w395
      frame 0, Default {
        n220 = local read "omega_y(M_avg)"() -> (w399:fxp<+/-,64,35>)
        n221 = local read "Dy_d (M_avg)"() -> (w398:fxp<+,64,32>)
      }
      frame 1 {
        n222 = local read "omega_y (M)"() -> (w400:fxp<+/-,64,30>)
        n223 = local read "Dy_d (M)"() -> (w401:fxp<+/-,64,27>)
      }
      frame 2 {
        n224 = local read "omega_y (T)"() -> (w403:fxp<+/-,20,9>)
        n225 = local read "Dy_d (T)"() -> (w402:fxp<+/-,46,10>)
      }
    }
    "omega_y (rad/s)" <- w396
    "Dy_d (mm/s)" <- w395
  }
  n226 = while "AO_y" {
    stop <- FALSE stop-if-true
    n227 = flat-sequence {
      frame #0 {
        n228 = local read "rad_y(NrTheta)"() -> (w416:fxp<+/-,48,33>)
        n229 = local read "vq_y"() -> (w419:fxp<+/-,20,5>)
        n230 = local read "vd_y"() -> (w418:fxp<+/-,20,5>)
        n231 = xnode "High Throughput Sine & Cosine"("x (pi)"=w416) -> ("sin(x)"=w412:fxp<+/-,16,2>, "cos(x)"=w411:fxp<+/-,16,2>)
        n232 = Select(t=fxp<+,1,1> 0.0, s="Stop motor_y", f=w419) -> (s? t:f=w414:fxp<+/-,20,5>)
        n233 = Select(t=fxp<+/-,20,5> 0.0, s="Stop motor_y", f=w418) -> (s? t:f=w413:fxp<+/-,20,5>)
        n234 = Negate(x=w414) -> (-x=w415:fxp<+/-,21,6>)
        n235 = Multiply(x=w413, y=w412) -> (x*y=w410:fxp<+/-,36,7>)
        n236 = Multiply(x=w413, y=w411) -> (x*y=w408:fxp<+/-,36,7>)
        n237 = Multiply(x=w411, y=w414) -> (x*y=w409:fxp<+/-,36,7>)
        n238 = Multiply(x=w412, y=w415) -> (x*y=w407:fxp<+/-,35,6>)
        n239 = Add(x=w410, y=w409) -> (x+y=→"vb_y":fxp<+/-,37,8>)
        n240 = Add(x=w408, y=w407) -> (x+y=→"va_y":fxp<+/-,36,7>)
      }
      frame #1 {
        n241 = local read "Encoder Reset_y"() -> (w462:bool)
        n242 = local read "va_y"() -> (w461:fxp<+/-,36,7>)
        n243 = local read "vb_y"() -> (w460:fxp<+/-,37,8>)
        n244 = Select(t=fxp<+/-,20,5> 5.0, s=w462, f=w461) -> (s? t:f=w457:fxp<+/-,36,7>)
        n245 = Select(t=fxp<+/-,20,5> 0.0, s=w462, f=w460) -> (s? t:f=w456:fxp<+/-,37,8>)
        n246 = Multiply(x=w456, y=fxp<+/-,20,5> -0.5) -> (x*y=w452:fxp<+/-,55,11>)
        n247 = Multiply(x=w457, y=fxp<+/-,20,5> -0.5) -> (x*y=w453:fxp<+/-,55,11>)
        n248 = xnode "FPGA I/O Node"("Mod8/AO2"=w453, "Mod8/AO3"=w452) -> ()  [unwired: 2 in, 2 out]
      }
    }
  }
  n249 = while "Quadrature drive_y" {
    stop <- FALSE stop-if-true
    n250 = local read "omega_y (rad/s)"() -> (w469:fxp<+/-,64,35>)
    n251 = local read "Fmr_y"() -> (w464:fxp<+/-,64,50>)
    n252 = call "Oriental_step_motor_PKP225.vi"("F_Threshold"=fxp<+,12,12> 10.0, "dFmr"=fxp<+/-,25,15> 0.0, "omega"=w469, "Fmr"=w464) -> ("vq_F"=→"vq_y":fxp<+/-,20,5>, "vd_F"=→"vd_y":fxp<+/-,20,5>)  [unwired: 6 in]
  }
  n253 = while "PID postition controller_y" {
    stop <- FALSE stop-if-true
    n254 = local read "Dy_i"() -> (w471:fxp<+/-,32,16>)
    n255 = local read "Dyr"() -> (w472:fxp<+/-,32,7>)
    n256 = local read "Dy (mm)"() -> (w481:fxp<+/-,56,32>)
    n257 = local read "Dy_dd"() -> (w482:fxp<+/-,36,47>)
    n258 = xnode "High Throughput Multiply"("x"="Ki_y", "y"=w471) -> ("x*y"=w480:fxp<+/-,48,17>)
    n259 = xnode "High Throughput Subtract"("x"=w472, "y"=w481) -> ("x-y"=w473:fxp<+/-,58,33>)
    "Dy_error" <- w473
    n260 = Absolute Value(x=w473) -> (abs(x)=w474:fxp<+,58,33>)
    n261 = Greater?(x=w474, y="Dy_tolorence") -> (0:w485:bool)
    n262 = Select(t=fxp<+,1,1> 1.0, s=w485, f=fxp<+,1,1> 0.0) -> (s? t:f=w488:fxp<+,1,1>)
    n263 = xnode "High Throughput Multiply"("x"=w473, "y"="Kp_y") -> ("x*y"=w479:fxp<+/-,64,34>)
    n264 = xnode "High Throughput Multiply"("x"=w482, "y"="Kd_y") -> ("x*y"=w478:fxp<+/-,52,48>)
    n265 = xnode "High Throughput Multiply"("x"=w480, "y"=w488) -> ("x*y"=w476:fxp<+/-,48,17>)
    n266 = xnode "High Throughput Add"("x"=w479, "y"=w478) -> ("x+y"=w477:fxp<+/-,64,49>)
    n267 = xnode "High Throughput Add"("x"=w477, "y"=w476) -> ("x+y"=→"Fmr_y":fxp<+/-,64,50>)
  }
  n268 = while "Time reset_y" {
    shift-right: [w497] -> _
    shift-left: _ -> [w496]
    shift-right: [w495] -> _
    shift-left: _ -> [w498]
    stop <- FALSE stop-if-true
    n269 = local read "Stop motor_y"() -> (w502:bool)
    n270 = call "Tick Count8"() -> ("Tick Count(uSec)"=w497:u32)
    n271 = Subtract(x=w497, y=w496) -> (x-y=w501:u32)
    n272 = Add(x=w498, y=w501) -> (x+y=w499:u32)
    n273 = Select(t=u32 0, s=w502, f=w499) -> (s? t:f=w495:u32)
    n274 = To Fixed-Point(number=w495) -> (fixed-point=w494:fxp<+,32,32>)  [unwired: 1 in]
    n275 = Multiply(x=fxp<+,20,-18> 1.0000003385357559e-06, y=w494) -> (x*y=→"Time now_y (s)":fxp<+,52,14>)
  }
  n276 = while "Command_y" {
    stop <- FALSE stop-if-true
    n277 = case shown="0, Default" "Command type_y" {
      tunnel: "Direction_y" -> [w510 w514 w517]
      tunnel: [w509 w511 w518] -> w504
      frame 0, Default {
        n278 = local read "Dyr_end"() -> (w507:fxp<+/-,32,7>)
        n279 = Negate(x=w507) -> (-x=w508:fxp<+/-,33,8>)
        n280 = Select(t=w507, s=w510, f=w508) -> (s? t:f=w509:fxp<+/-,33,8>)
      }
      frame 1 {
        n281 = local read "Dyr_ramp"() -> (w512:fxp<+/-,32,7>)
        n282 = Negate(x=w512) -> (-x=w513:fxp<+/-,33,8>)
        n283 = Select(t=w512, s=w514, f=w513) -> (s? t:f=w511:fxp<+/-,33,8>)
      }
      frame 2 {
        n284 = local read "Dyr_sin"() -> (w515:fxp<+/-,30,11>)
        n285 = Negate(x=w515) -> (-x=w516:fxp<+/-,29,10>)
        n286 = Select(t=w515, s=w517, f=w516) -> (s? t:f=w518:fxp<+/-,30,11>)
      }
    }
    "Dyr" <- w504
  }
  n287 = while "Stroke_y" {
    stop <- FALSE stop-if-true
    n288 = local read "Command type_y"() -> (w520:i16)
    n289 = case shown="0, Default" w520 {
      frame 0, Default {
        n290 = while "Step" {
          stop <- w522 stop-if-true
          n291 = local read "Dy (mm)"() -> (w527:fxp<+/-,56,32>)
          n292 = local read "Dy_tolorence"() -> (w525:fxp<+/-,18,1>)
          n293 = local read "Dyr_end"() -> (w521:fxp<+/-,32,7>)
          n294 = Absolute Value(x=w527) -> (abs(x)=w526:fxp<+,56,32>)
          n295 = Subtract(x=w526, y=w525) -> (x-y=w524:fxp<+/-,57,33>)
          n296 = Absolute Value(x=w521) -> (abs(x)=w523:fxp<+,32,7>)
          n297 = Greater Or Equal?(x=w524, y=w523) -> (x >= y?=w522:bool)
          n298 = case shown="True" w522 {
            selector: w522 -> [_ w528]
            frame False {
            }
            frame True {
              n299 = local write "Stop motor_y"(w528) -> ()
            }
          }
        }
      }
      frame 1 {
        n300 = while "Ramp" {
          stop <- w529 stop-if-true
          n301 = local read "Dy (mm)"() -> (w533:fxp<+/-,56,32>)
          n302 = local read "Dy_tolorence"() -> (w532:fxp<+/-,18,1>)
          n303 = local read "Dyr_end"() -> (w530:fxp<+/-,32,7>)
          n304 = Absolute Value(x=w533) -> (abs(x)=w534:fxp<+,56,32>)
          n305 = Subtract(x=w534, y=w532) -> (x-y=w531:fxp<+/-,57,33>)
          n306 = Greater Or Equal?(x=w531, y=w530) -> (x >= y?=w529:bool)
          n307 = case shown="True" w529 {
            selector: w529 -> [_ w535]
            frame False {
            }
            frame True {
              n308 = local write "Stop motor_y"(w535) -> ()
            }
          }
        }
      }
      frame 2 {
      }
    }
  }
  n309 = while "omega_y (M_avg)" {
    tunnel: w4 -> [w545]
    tunnel: w3 -> [w551]
    shift-right: [w541] -> _
    shift-left: w1 -> [w542]
    shift-right: [w540] -> _
    shift-left: w2 -> [w546]
    shift-right: [w538] -> _
    shift-left: _ -> [w543]
    stop <- FALSE stop-if-true
    w539 = fxp<+/-,27,3> 3.1415926218032837  # pi
    n310 = Multiply(x=w545, y=w551) -> (x*y=w550:u32)
    n311 = Index Array(array=w542, index=0) -> (element=w547:u32)
    n312 = Index Array(array=w546, index=0) -> (element=w544:i32)
    n313 = call "Tick Count5"() -> ("Tick Count(uSec)"=w548:u32)
    n314 = Add(x=w550, y=w547) -> (x+y=w554:u32)
    n315 = Greater Or Equal?(x=w548, y=w554) -> (x >= y?=w549:bool)
    n316 = case shown="True" w549 {
      tunnel: w548 -> [_ w577]
      tunnel: w547 -> [_ w578]
      tunnel: w546 -> [w556 w567]
      tunnel: w545 -> [_ w568]
      tunnel: w544 -> [_ w569]
      tunnel: w543 -> [w555 _]
      tunnel: w542 -> [w557 w579]
      tunnel: [w557 w560] -> w541
      tunnel: [w556 w559] -> w540
      tunnel: [w555 w558] -> w538
      frame False {
      }
      frame True {
        n317 = local read "Encoder Position_y"() -> (w570:i32)
        n318 = Subtract(x=w577, y=w578) -> (x-y=w576:u32)
        n319 = To Fixed-Point(number=w576) -> (fixed-point=w575:fxp<+,32,32>)  [unwired: 1 in]
        n320 = Subtract(x=w570, y=w569) -> (x-y=w571:i32)
        n321 = Multiply(x=w571, y=u32 2500) -> (x*y=w573:u32)
        n322 = Insert Into Array(array=w579, new element=w577) -> (w565:u32[])  [unwired: 1 in]
        n323 = Insert Into Array(array=w567, index=w568, new element=w570) -> (w566:i32[])
        n324 = To Fixed-Point(number=w573) -> (fixed-point=w574:fxp<+,32,32>)  [unwired: 1 in]
        n325 = Divide(x=w574, y=w575) -> (x/y=w558:fxp<+,64,32>)
        n326 = Delete From Array(array=w565, length=1, index=0) -> (array with subset deleted=w560:u32[])  [unwired: 1 out]
        n327 = Delete From Array(array=w566, length=1, index=0) -> (array with subset deleted=w559:i32[])  [unwired: 1 out]
      }
    }
    "Dy_d (M_avg)" <- w538
    n328 = Multiply(x=w539, y=w538) -> (x*y=→"omega_y(M_avg)":fxp<+/-,64,35>)
  }
  n329 = while "Integral and derivative_y" {
    shift-right: [w601] -> _
    shift-left: _ -> [w604]
    shift-right: [w590] -> _
    shift-left: _ -> [w581]
    shift-right: [w583] -> _
    shift-left: _ -> [w582]
    stop <- FALSE stop-if-true
    n330 = local read "Dy (mm)"() -> (w601:fxp<+/-,56,32>)
    n331 = local read "Dy_tolorence"() -> (w596:fxp<+/-,18,1>)
    n332 = local read "Dy_error"() -> (w593:fxp<+/-,57,33>)
    n333 = Subtract(x=w601, y=w604) -> (x-y=w603:fxp<+/-,57,33>)
    n334 = Absolute Value(x=w593) -> (abs(x)=w597:fxp<+,57,33>)
    n335 = Multiply(x=w603, y=fxp<+,7,10> 1000.0) -> (x*y=w600:fxp<+/-,64,43>)
    n336 = Greater?(x=w597, y=w596) -> (0:w595:bool)
    n337 = local read "Stop motor_y"() -> (w587:bool)
    n338 = Select(t=w593, s=w595, f=fxp<+,24,11> 0.0) -> (s? t:f=w590:fxp<+/-,57,33>)
    n339 = xnode "Butterworth Filter"("input data"=w600, "scaled coefficients"="scaled coefficients_Dy_dd") -> ("output data"=→"Dy_dd":fxp<+/-,36,47>)  [unwired: 1 in]
    n340 = Add(x=w581, y=w590) -> (x+y=w592:fxp<+/-,58,34>)
    n341 = Multiply(x=fxp<+/-,30,12> 0.000499725341796875, y=w592) -> (x*y=w589:fxp<+/-,64,46>)
    n342 = Select(t=fxp<+,1,1> 0.0, s=w587, f=fxp<+,1,1> 1.0) -> (s? t:f=w584:fxp<+,1,1>)
    n343 = Add(x=w589, y=w582) -> (x+y=w588:fxp<+/-,32,16>)
    n344 = Multiply(x=w588, y=w584) -> (x*y=w583:fxp<+/-,32,16>)
    "Dy_i" <- w583
    n345 = call "Wait4"("Count(uSec)"=u32 1000) -> ()  [unwired: 1 out]
  }
  n346 = while "Encoder_y" {
    shift-right: [w622] -> _
    shift-left: _ -> [w620]
    shift-right: [w623] -> _
    shift-left: _ -> [w621]
    shift-right: [w626] -> _
    shift-left: _ -> [w625]
    stop <- FALSE stop-if-true
    n347 = xnode "FPGA I/O Node"() -> ("Mod4/DI0"=w627:bool, "Mod4/DI1"=w628:bool)  [unwired: 2 in, 2 out]
    n348 = call "encoder_sub.vi"("A_pre"=w620, "B_pre"=w621, "Encoder Position_pre"=w625, "A input"=w627, "Encoder Position Reset"="Encoder Reset_y", "B input"=w628) -> ("A"=w622:bool, "B"=w623:bool, "Encoder Position (Counts)"=w626:i32)  [unwired: 19 in]
    "Encoder Position_y" <- w626
    n349 = To Fixed-Point(number=w626) -> (fixed-point=w617:fxp<+/-,32,32>)  [unwired: 1 in]
    n350 = xnode "High Throughput Multiply"("x"=w617, "y"=fxp<+/-,24,0> 0.002499997615814209) -> ("x*y"=→"Dy (mm)":fxp<+/-,56,32>)
    n351 = xnode "High Throughput Multiply"("x"=w617, "y"=fxp<+/-,16,1> 0.125) -> ("x*y"=→"rad_y(NrTheta)":fxp<+/-,48,33>)
  }
  n352 = while {
    stop <- FALSE stop-if-true
    w644 = fxp<+,20,3> 6.2831878662109375  # 2*pi
    n353 = local read "Time now_y (s)"() -> (w651:fxp<+,52,14>)
    n354 = Multiply(x=fxp<+,1,2> 2.0, y="Sin wave frequency_y (Hz)") -> (x*y=w650:fxp<+/-,21,6>)
    n355 = local read "Sin wave frequency_y (Hz)"() -> (w643:fxp<+/-,21,5>)
    n356 = Multiply(x=w650, y=w651) -> (x*y=w652:fxp<+/-,64,20>)
    n357 = local read "Sin magnitude_y"() -> (w642:fxp<+/-,11,8>)
    n358 = local read "Sin magnitude_y"() -> (w637:fxp<+/-,11,8>)
    n359 = local read "Sin omega_y"() -> (w638:fxp<+/-,41,8>)
    n360 = xnode "High Throughput Sine & Cosine"("x (pi)"=w652) -> ("sin(x)"=w635:fxp<+/-,18,2>, "cos(x)"=w639:fxp<+/-,18,2>)
    n361 = Square(x=w638) -> (x^2=w646:fxp<+,64,14>)
    n362 = Multiply(x=w644, y=w643) -> (x*y=w641:fxp<+/-,41,8>)
    "Sin omega_y" <- w641
    n363 = Negate(x=w646) -> (-x=w645:fxp<+/-,64,15>)
    n364 = Multiply(x=w641, y=w642) -> (x*y=w640:fxp<+/-,51,15>)
    n365 = Multiply(x=w645, y=w637) -> (x*y=w636:fxp<+/-,64,23>)
    n366 = Multiply(x=w639, y=w640) -> (x*y=→"Dyr_sin_d":fxp<+/-,64,16>)
    n367 = Multiply(x=w635, y=w636) -> (x*y=→"Dyr_sin_dd":fxp<+/-,64,25>)
    n368 = Multiply(x="Sin magnitude_y", y=w635) -> (x*y=w634:fxp<+/-,29,10>)
    n369 = Add(x=w634, y="Sin offset_y") -> (x+y=→"Dyr_sin":fxp<+/-,30,11>)
  }
  n370 = while "Ramp gene._y" {
    stop <- FALSE stop-if-true
    n371 = flat-sequence {
      frame #0 {
        n372 = Divide(x="Dyr_end", y="Dyr_time") -> (x/y=→"Dyr_slope":fxp<+/-,64,30>)
      }
      frame #1 {
        n373 = local read "Time now_y (s)"() -> (w687:fxp<+,52,14>)
        n374 = while {
          tunnel: w687 -> [w692]
          stop <- FALSE stop-if-true
          n375 = local read "Time now_y (s)"() -> (w693:fxp<+,52,14>)
          n376 = local read "Dyr_slope"() -> (w690:fxp<+/-,32,10>)
          n377 = Subtract(x=w693, y=w692) -> (x-y=w691:fxp<+/-,53,15>)
          n378 = Multiply(x=w690, y=w691) -> (x*y=→"Dyr_ramp":fxp<+/-,64,24>)
        }
      }
    }
  }
